vi "PCO_ConvertGetDisplay.vi"(8 "error in (no error)":errorcluster {"code" format="%x"}, 11 "ph":u64) -> (0 "error out":errorcluster {"code" format="%x"}, 1 "strDisplay":T1, 2 "ErrorMessage":i32 format="%x", 3 "ph out":u64)   [LabVIEW 2019, in "Convert.lvlib"]
doc: "int PCOCONVERT_API PCO_ConvertGetDisplay(HANDLE ph, PCO_Display* pstrDisplay);"
uses:
  Convert.lvlib
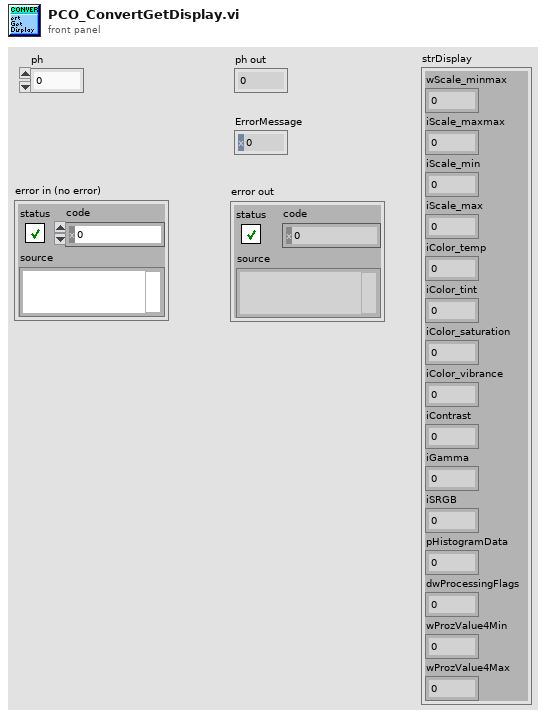
[diagram p1: front panel]
types:
  T1 = cluster{"wScale_minmax":u16, "iScale_maxmax":i32, "iScale_min":i32, "iScale_max":i32, "iColor_temp":i32, "iColor_tint":i32, "iColor_saturation":i32, "iColor_vibrance":i32, "iContrast":i32, "iGamma":i32, "iSRGB":i32, "pHistogramData":u64, "dwProcessingFlags":u32, "wProzValue4Min":u16, "wProzValue4Max":u16}
  T2 = cluster{"wSize":u16, "wScale_minmax":u16, "iScale_maxmax":i32, "iScale_min":i32, "iScale_max":i32, "iColor_temp":i32, "iColor_tint":i32, "iColor_saturation":i32, "iColor_vibrance":i32, "iContrast":i32, "iGamma":i32, "iSRGB":i32, "pHistogramData":u64, "dwDialogOpenFlags":u32, "dwProcessingFlags":u32, "wProzValue4Min":u16, "wProzValue4Max":u16, "dwzzDummy1":cluster{u32, u32, u32, u32, u32, u32, u32, u32, u32, u32, u32, u32, u32, u32, u32, u32, u32, u32, u32, u32, u32, u32, u32, u32, u32, u32, u32, u32, u32, u32, u32, u32, u32, u32, u32, u32, u32, u32, u32, u32, u32, u32, u32, u32, u32, u32, u32, u32, u32, u32}}
  T3 = cluster{"wSize":u16, "wScale_minmax":u16, "iScale_maxmax":i32, "iScale_min":i32, "iScale_max":i32, "iColor_temp":i32, "iColor_tint":i32, "iColor_saturation":i32, "iColor_vibrance":i32, "iContrast":i32, "iGamma":i32, "iSRGB":i32, "pHistogramData":u32, "dwDialogOpenFlags":u32, "dwProcessingFlags":u32, "wProzValue4Min":u16, "wProzValue4Max":u16, "dwzzDummy1":cluster{u32, u32, u32, u32, u32, u32, u32, u32, u32, u32, u32, u32, u32, u32, u32, u32, u32, u32, u32, u32, u32, u32, u32, u32, u32, u32, u32, u32, u32, u32, u32, u32, u32, u32, u32, u32, u32, u32, u32, u32, u32, u32, u32, u32, u32, u32, u32, u32, u32}}
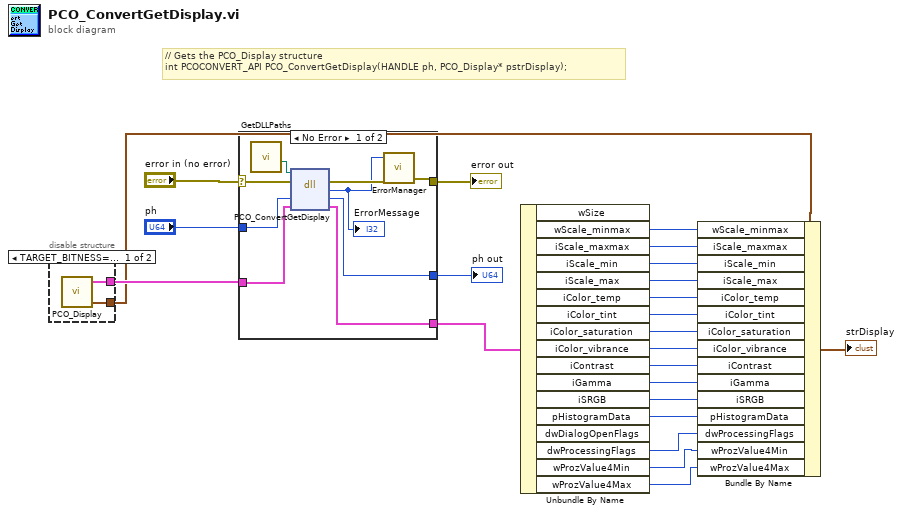
[diagram p0: block diagram]
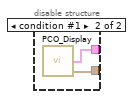
[diagram p2: hidden frame]
diagram:
  # "// Gets the PCO_Display structure\nint PCOCONVERT_API PCO_ConvertGetDisplay(HANDLE ph, PCO_Display* pstrDisplay);"
  n1 = disable-structure "Diagram Disable Structure" shown="TARGET_BITNESS==64, Default" {
    disable-tunnel: [w25 w27] -> w19
    disable-tunnel: [w24 w26] -> w17
    frame condition #0 (active) {
      n2 = call "PCO_Display.vi"() -> ("PCO_DisplayRaw_x64"=w25:T2, "PCO_Display"=w24:T1)  [unwired: 4 in, 3 out]
    }
    frame condition #1 {
      n3 = call "PCO_Display.vi"() -> ("PCO_DisplayRaw_win32"=w27:T3, "PCO_Display"=w26:T1)  [unwired: 4 in, 3 out]
    }
  }
  n4 = case shown="No Error" "error in (no error)" {
    selector: "error in (no error)" -> [w33 w39]
    tunnel: "ph" -> [w36 w38]
    tunnel: [w35 w38] -> w22
    tunnel: [w34 w37] -> w18
    tunnel: [w31 w39] -> w21
    tunnel: w19 -> [w29 w37]
    frame No Error {
      n5 = call "GetDLLPaths.vi"() -> ("PCO_Conv_Path"=w28:path)  [unwired: 9 in, 2 out]
      n6 = dll-call lib="?" fn="PCO_ConvertGetDisplay"(path in=w28, error in=w33, "ph"=w36, "pstrDisplay"=w29) -> (error out=w32:errorcluster, "return type"=w30:i32, "ph"=w35:u64, "pstrDisplay"=w34:T2)  [unwired: 1 in, 1 out]
      "ErrorMessage" <- w30
      n7 = call "ErrorManager.vi"("error in (no error)"=w32, "error code"=w30) -> ("error out"=w31:errorcluster)  [unwired: 3 in]
    }
    frame Error {
    }
  }
  "ph out" <- w22
  "error out" <- w21
  n8 = Unbundle By Name(w18) -> ("wScale_minmax"=w16:u16, "iScale_maxmax"=w15:i32, "iScale_min"=w14:i32, "iScale_max"=w13:i32, "iColor_temp"=w12:i32, "iColor_tint"=w11:i32, "iColor_saturation"=w10:i32, "iColor_vibrance"=w9:i32, "iContrast"=w8:i32, "iGamma"=w7:i32, "iSRGB"=w6:i32, "pHistogramData"=w5:u64, "dwProcessingFlags"=w4:u32, "wProzValue4Min"=w3:u16, "wProzValue4Max"=w2:u16)  [unwired: 2 out]
  n9 = Bundle By Name(cluster=w17, "wScale_minmax"=w16, "iScale_maxmax"=w15, "iScale_min"=w14, "iScale_max"=w13, "iColor_temp"=w12, "iColor_tint"=w11, "iColor_saturation"=w10, "iColor_vibrance"=w9, "iContrast"=w8, "iGamma"=w7, "iSRGB"=w6, "pHistogramData"=w5, "dwProcessingFlags"=w4, "wProzValue4Min"=w3, "wProzValue4Max"=w2) -> (→"strDisplay":T1)
